vi "SNtoIDCHKSUM(SubVI).vi"(10 "fix cheksum":u8, 11 "input sn":string) -> (1 "output check sum":u8, 2 "output sn":string, 3 "output id":u8 format="%x")   [LabVIEW 2012]
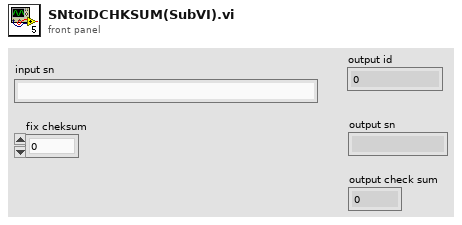
[diagram p1: front panel]
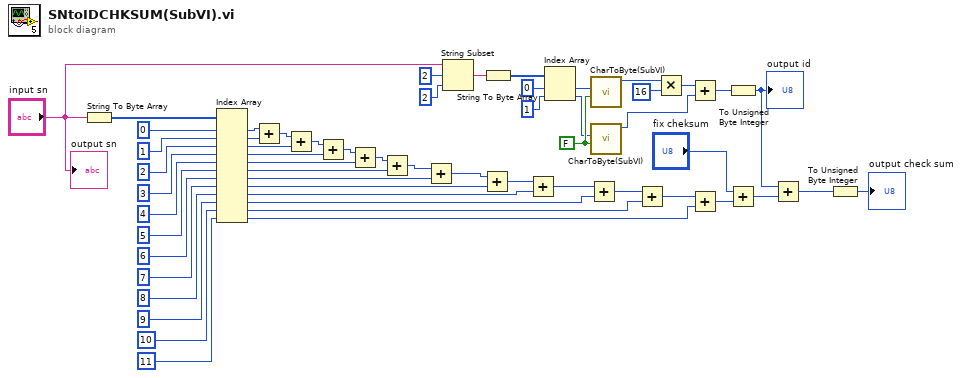
[diagram p0: block diagram]
diagram:
  w50 = FALSE
  n1 = String To Byte Array(string="input sn") -> (unsigned byte array=w40:u8[])
  n2 = Index Array(array=w40, index #1=0, index #2=1, index #3=2, index #4=3, index #5=4, index #6=5, index #7=6, index #8=7, index #9=8, index #10=9, index #11=10, index #12=11) -> (element #1=w27:u8, element #2=w26:u8, element #3=w24:u8, element #4=w22:u8, element #5=w2:u8, element #6=w3:u8, element #7=w4:u8, element #8=w5:u8, element #9=w6:u8, element #10=w7:u8, element #11=w8:u8, element #12=w9:u8)
  n3 = Add(x=w27, y=w26) -> (x+y=w25:u8)
  n4 = Add(x=w25, y=w24) -> (x+y=w23:u8)
  n5 = Add(x=w23, y=w22) -> (x+y=w21:u8)
  n6 = Add(x=w21, y=w2) -> (x+y=w20:u8)
  n7 = Add(x=w20, y=w3) -> (x+y=w19:u8)
  n8 = Add(x=w19, y=w4) -> (x+y=w18:u8)
  n9 = String Subset(string="input sn", offset (0)=2, length (rest)=2) -> (substring=w44:string)
  n10 = Add(x=w18, y=w5) -> (x+y=w17:u8)
  n11 = String To Byte Array(string=w44) -> (unsigned byte array=w45:u8[])
  n12 = Add(x=w17, y=w6) -> (x+y=w16:u8)
  n13 = Index Array(array=w45, index #1=0, index #2=1) -> (element #1=w48:u8, element #2=w49:u8)
  n14 = Add(x=w16, y=w7) -> (x+y=w15:u8)
  n15 = call "CharToByte(SubVI).vi"("use char"=w50, "input u8"=w48) -> ("output u8"=w51:u8)  [unwired: 7 in, 2 out]
  n16 = call "CharToByte(SubVI).vi"("use char"=w50, "input u8"=w49) -> ("output u8"=w52:u8)  [unwired: 7 in, 2 out]
  n17 = Add(x=w15, y=w8) -> (x+y=w14:u8)
  n18 = Multiply(x=w51, y=16) -> (x*y=w53:i32)
  n19 = Add(x=w53, y=w52) -> (x+y=w55:i32)
  n20 = Add(x=w14, y=w9) -> (x+y=w12:u8)
  n21 = To Unsigned Byte Integer(number=w55) -> (unsigned 8bit integer=w1:u8)
  "output id" <- w1
  n22 = Add(x="fix cheksum", y=w12) -> (x+y=w11:u8)
  n23 = Add(x=w1, y=w11) -> (x+y=w10:u8)
  n24 = To Unsigned Byte Integer(number=w10) -> (unsigned 8bit integer=→"output check sum":u8)
  "output sn" <- "input sn"
